vi "ITXtoTDMS.vi"(11 "Currrent ITX file 2":path) -> ()   [LabVIEW 2016]
uses:
  <userlib>/LevyLab/LV to ITX/LVtoITX.lvclass
panel:
  out "parseable data":string
  # "Manually add values that were not recorded but are known"
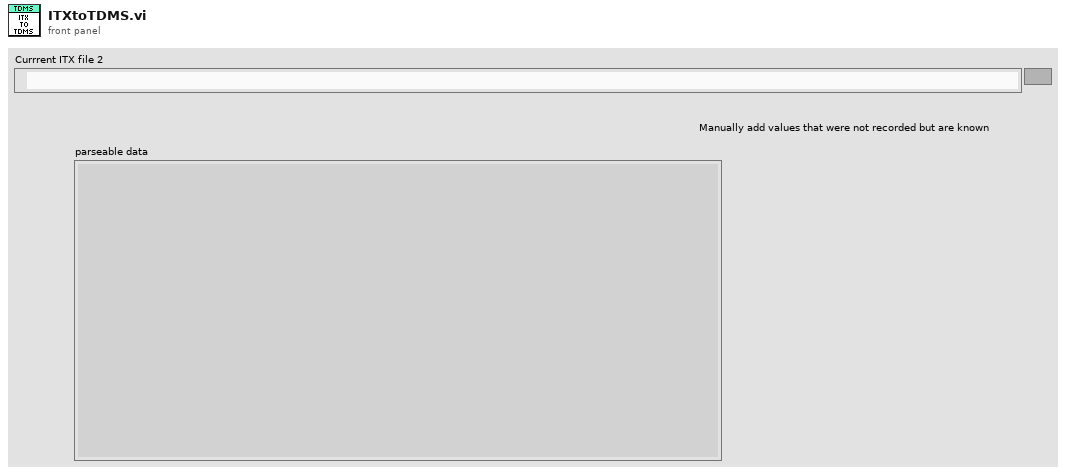
[diagram p1: front panel]
types:
  T1 = enum16{"open", "open or create", "create or replace", "create", "open (read-only)"}
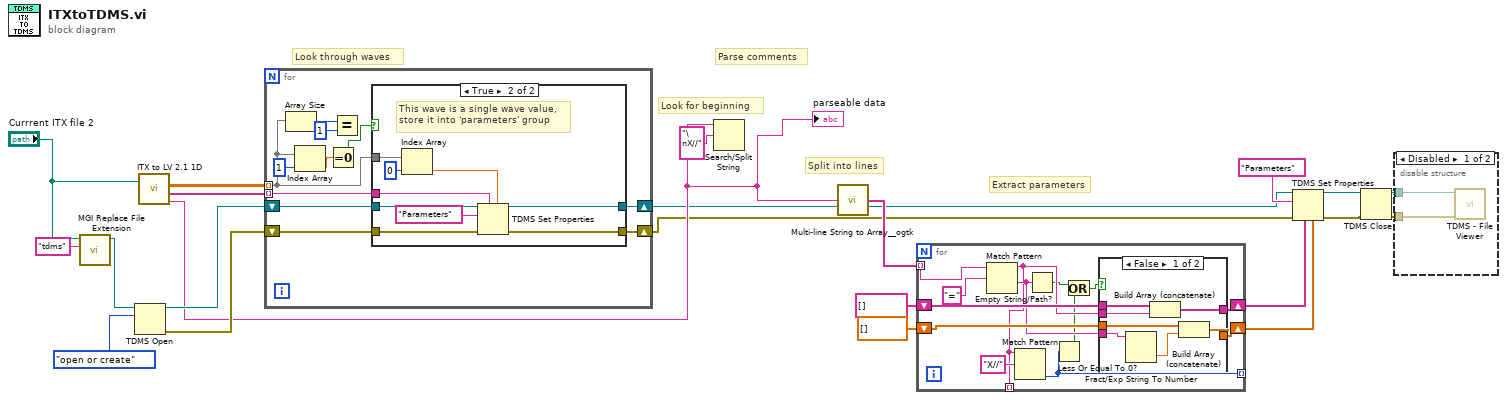
[diagram p0: block diagram]
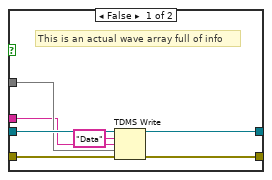
[diagram p4: hidden frame]
diagram:
  # "Extract parameters"
  # "Look for beginning"
  # "Split into lines"
  # "Parse comments"
  # "Look through waves"
  n1 = call <userlib>:"MGI Replace File Extension.vi"("New Extension (txt)"="tdms", "Path In"="Currrent ITX file 2") -> ("Path Out"=w18:path)  [unwired: 8 in, 1 out]
  n2 = TDMS Open(10:T1."open or create" ("operation (0:open)"), 11:w18) -> (0:w14:errorcluster, 3:w15:refnum<k34>)  [unwired: 5 in]
  n3 = call <userlib>:"ITX to LV 2.1 1D.vi"("file (use dialog)"="Currrent ITX file 2") -> ("1D arrays"=w17:dbl[][], "wave names"=w16:string[], "Notes"=w11:string)  [unwired: 2 in]
  "parseable data" <- w11
  n4 = for {
    tunnel: w17 -> [w26] mode=indexing
    tunnel: w16 -> [w31] mode=indexing
    shift-right: [w30] -> w4
    shift-left: w15 -> [w32]
    shift-right: [w28] -> w3
    shift-left: w14 -> [w29]
    n5 = Array Size(array=w26) -> (size(s)=w27:i32)
    n6 = Index Array(array=w26, index=1) -> (element=w24:dbl)
    n7 = Equal To 0?(x=w24) -> (x = 0?=w23:bool)
    n8 = Equal?(x=w27, y=1) -> ()  [unwired: 1 out]
    n9 = case shown="True" w23 {
      tunnel: w26 -> [w37 w49]
      tunnel: w32 -> [w40 w47]
      tunnel: w31 -> [w36 w45]
      tunnel: [w39 w43] -> w30
      tunnel: w29 -> [w35 w41]
      tunnel: [w34 w42] -> w28
      frame False {
        # "This is an actual wave array full of info"
        n10 = TDMS Write(0:w40, 5:"Data" ("group name in (Untitled)"), 7:w36, 9:w37, 11:w35) -> (4:w39:refnum<k34>, 15:w34:errorcluster)  [unwired: 1 in, 2 out]
      }
      frame True {
        # "This wave is a single wave value,\nstore it into 'parameters' group"
        n11 = Index Array(array=w49, index=0) -> (element=w44:dbl)
        n12 = TDMS Set Properties(5:w44, 7:w45, 8:w41, 10:"Parameters" ("group name"), 11:w47) -> (0:w42:errorcluster, 3:w43:refnum<k34>)  [unwired: 1 in, 2 out]
      }
    }
  }
  n13 = Search/Split String(string=w11, search string/char (-)="\nX//") -> ()  [unwired: 1 in, 3 out]
  n14 = call <userlib>:"Multi-line String to Array__ogtk.vi"("string"=w11) -> ("lines"=w10:string[])
  n15 = for {
    tunnel: w10 -> [w62] mode=indexing
    shift-right: [w59] -> w6
    shift-left: string[] [] -> [w60]
    shift-right: [w58] -> w5
    shift-left: dbl[] [] -> [w57]
    tunnel: [w53] -> _ mode=indexing
    tunnel: [w54] -> _ mode=indexing
    n16 = Match Pattern(string=w62, regular expression="=") -> (before substring=w54:string, after substring=w55:string)  [unwired: 1 in, 2 out]
    n17 = Match Pattern(string=w54, regular expression="X//") -> (offset past match=w53:i32)  [unwired: 1 in, 3 out]
    n18 = Empty String/Path?(string/path=w55) -> (empty?=w51:bool)
    n19 = Less Or Equal To 0?(x=w53) -> (x <= 0?=w52:bool)
    n20 = Or(x=w51, y=w52) -> (x .or. y?=w50:bool)
    n21 = case shown="False" w50 {
      tunnel: w55 -> [w64 _]
      tunnel: w54 -> [w69 _]
      tunnel: w60 -> [w68 w71]
      tunnel: [w67 w71] -> w59
      tunnel: [w66 w70] -> w58
      tunnel: w57 -> [w65 w70]
      frame False {
        n22 = Fract/Exp String To Number(string=w64) -> (number=w63:dbl)  [unwired: 3 in, 1 out]
        n23 = Build Array (concatenate)(w68, w69) -> (w67:string[])
        n24 = Build Array (concatenate)(w65, w63) -> (w66:dbl[])
      }
      frame True {
      }
    }
  }
  n25 = TDMS Set Properties(5:w5, 7:w6, 8:w3, 10:"Parameters" ("group name"), 11:w4) -> (0:w2:errorcluster, 3:w1:refnum<k34>)  [unwired: 1 in, 2 out]
  n26 = TDMS Close(8:w2, 11:w1) -> (0:w20:errorcluster, 3:w21:path)
  n27 = disable-structure shown="Disabled" {
    disable-tunnel: w21 -> [w73 _]
    disable-tunnel: w20 -> [w72 _]
    frame Disabled {
      n28 = call <vilib>:"TDMS - File Viewer.vi"("error in (no error)"=w72, "file path"=w73) -> ()  [unwired: 4 in, 2 out]
    }
    frame Enabled {
    }
  }
